vi "globals.vi"() -> ()   [LabVIEW 2019]
panel:
  out "elapsed (min)":dbl
  out "BAT 2 V":u16
  out "BAT 1 V":u16
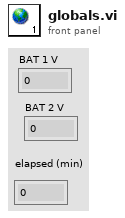
[diagram p1: front panel]
diagram:
